vi "replaceObjectPlaceHolders_const.vi"(7 "placeholderList":T1(array[cluster]), 8 "error in (no error)":errorcluster, 10 "targetVI":path, 11 "classPathToReplace":path) -> (0 "error out":errorcluster)   [LabVIEW 2023]
uses:
  <vilib>/Utility/traverseref.llb/TRef TravTarget.ctl
  <vilib>/Utility/traverseref.llb/VI Scripting - Traverse.lvlib
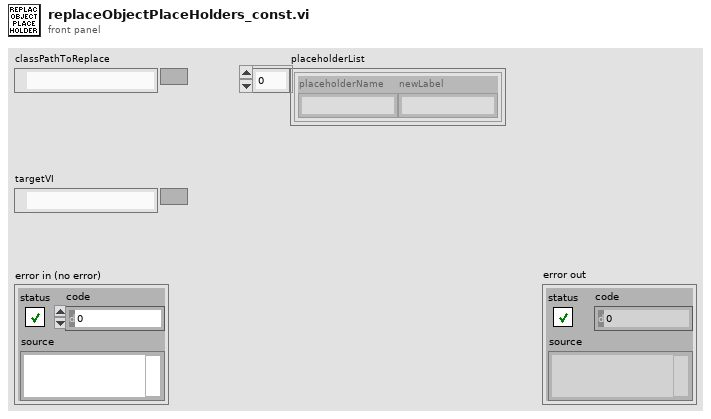
[diagram p1: front panel]
types:
  T1 = cluster{"placeholderName":string, "newLabel":string}[]
  T2 = typedef "TRef TravTarget.ctl" = enum16{"FP", "BD", "Other"}
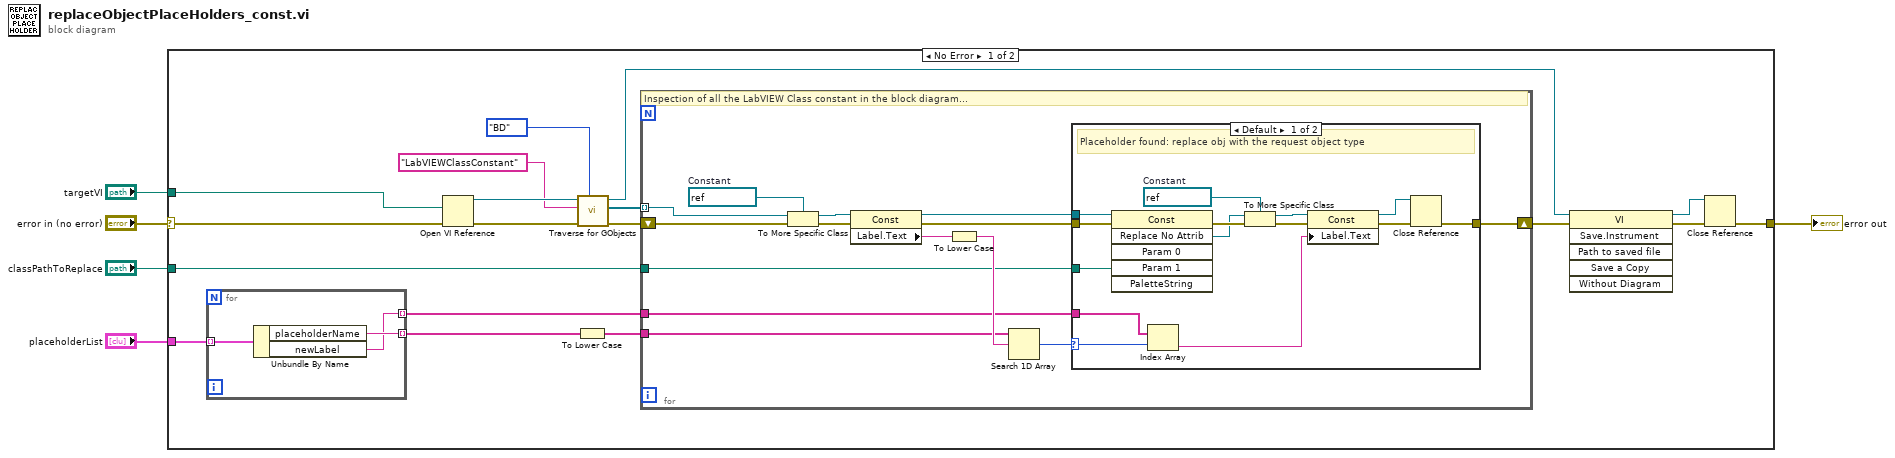
[diagram p0: block diagram]
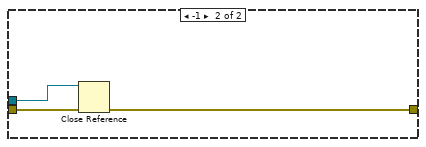
[diagram p2: hidden frame]
diagram:
  n1 = case shown="No Error" "error in (no error)" {
    selector: "error in (no error)" -> [w23 w58]
    tunnel: "classPathToReplace" -> [w18 _]
    tunnel: [w15 w58] -> w3
    tunnel: "placeholderList" -> [w13 _]
    tunnel: "targetVI" -> [w11 _]
    frame No Error {
      n2 = for {
        tunnel: w13 -> [w26] mode=indexing
        tunnel: [w25] -> w14 mode=indexing
        tunnel: [w24] -> w12 mode=indexing
        n3 = Unbundle By Name(w26) -> ("placeholderName"=w25:string, "newLabel"=w24:string)
      }
      n4 = Open VI Reference(vi path=w11, error in (no error)=w23) -> (vi reference=w22:refnum<vi>, error out=w21:errorcluster)  [unwired: 4 in]
      n5 = To Lower Case(string=w14) -> (all lower case string=w17:string[])
      n6 = call <vilib>:"Traverse for GObjects.vi"("Traverse Target"=TRef_TravTarget."BD", "error in (no error)"=w21, "Class Name"="LabVIEWClassConstant", "VI Refnum"=w22) -> ("error out"=w16:errorcluster, "References"=w10:refnum<vi>[], "dup VI Refnum"=w7:refnum<vi>)  [unwired: 4 in, 1 out]
      n7 = for {
        tunnel: w10 -> [w30] mode=indexing
        tunnel: w17 -> [w36]
        tunnel: w18 -> [w34]
        shift-right: [w27] -> w9
        shift-left: w16 -> [w32]
        tunnel: w12 -> [w29]
        w40 = refnum<vi> refnum  # Constant
        # "Inspection of all the LabVIEW Class constant in the block diagram..."
        n8 = To More Specific Class(target class=w40, reference=w30, error in=w32) -> (specific class reference=w39:refnum<vi>, error out=w33:errorcluster)
        n9 = property class="Const"(reference=w39, error in=w33) -> (reference out=w28:refnum<vi>, error out=w31:errorcluster, "Label.Text"=w38:string)
        n10 = To Lower Case(string=w38) -> (all lower case string=w37:string)
        n11 = Search 1D Array(1D array=w36, element=w37) -> (index of element=w35:i32)  [unwired: 1 in]
        n12 = case shown="Default" w35 {
          selector: w35 -> [w43 _]
          tunnel: w34 -> [w54 _]
          tunnel: w28 -> [w53 w55]
          tunnel: w31 -> [w52 w56]
          tunnel: [w44 w57] -> w27
          tunnel: w29 -> [w41 _]
          frame Default {
            w51 = refnum<vi> refnum  # Constant
            # "Placeholder found: replace obj with the request object type"
            n13 = invoke class="Const" method="Replace No Attrib"(reference=w53, error in=w52, "Param 1"=w54) -> (error out=w50:errorcluster, "RepNoAttrib"=w48:refnum<vi>)  [unwired: 3 in, 4 out]
            n14 = Index Array(array=w41, index=w43) -> (element=w42:string)
            n15 = To More Specific Class(target class=w51, reference=w48, error in=w50) -> (specific class reference=w47:refnum<vi>, error out=w49:errorcluster)
            n16 = property class="Const"(reference=w47, error in=w49, "Label.Text"=w42) -> (reference out=w46:refnum<vi>, error out=w45:errorcluster)
            n17 = Close Reference(reference=w46, error in (no error)=w45) -> (error out=w44:errorcluster)
          }
          frame -1 {
            n18 = Close Reference(reference=w55, error in (no error)=w56) -> (error out=w57:errorcluster)
          }
        }
      }
      n19 = invoke class="VI" method="Save.Instrument"(reference=w7, error in=w9) -> (reference out=w6:refnum<vi>, error out=w8:errorcluster)  [unwired: 4 in, 4 out]
      n20 = Close Reference(reference=w6, error in (no error)=w8) -> (error out=w15:errorcluster)
    }
    frame Error {
    }
  }
  "error out" <- w3
